vi "Config.View.vi"() -> ()   [LabVIEW 2019]
uses:
  Telas.ctl
  <vilib>/Utility/miscctls.llb/LVPositionTypeDef.ctl
  <vilib>/Utility/miscctls.llb/LVPointTypeDef.ctl
  TelaConfig/Configuracao.Variaveis.vi
panel:
  in  "NovaSenhaOk":bool
  out "SemSenha":bool
  out "SenhaCadastrada":i32[](array[numeric])
  out "ProximaTela":T1
  in  "Tab":enum32{"Page 1", "Page 2"}(tab)
  in  "Salvar":bool
  in  "TabTela":enum32{"Senha", "Campos1", "Campos2"}(tab)
  in  "NextSenha":bool
  out "AlertaSenha":string
  in  "Senha":string caption="SENHA"
  out "TexSegundo":string
  in  "ProximaTela":bool
  in  "AddParametro":bool caption="Adicionar:"
  in  "ListParamentos":string[][](table)
  in  "MeCompleta":bool caption="Memória completa:"
  in  "PosiçaoMemoria":dbl caption="Posiçao na memória:"
  out "TexBit":string
  in  "TamanhoMemoria":enum16{"1 bit", "8 bit", "16 bit"}(ring) caption="Tamanho:"
  in  "TipoMemoria":enum16{"Int", "Boleano"}(ring) caption="Tipo:"
  in  "Memoria":string caption="Memória:"
  in  "AceleracaoMaxima":dbl caption="Tempo mím aceleração:"
  in  "ModeloInversor":string caption="Modelo:"
  out "TexInversor":string
  in  "Parametros":T2(ring) caption="Parâmetros:"
  out "TexMotor":string
  in  "RotacaoMaxMotor":dbl caption="Rotação máxima:"
  in  "PotenciaMotor":dbl caption="Potência:"
  in  "ModeloMotor":string caption="Modelo:"
  in  "NovaSenha":string caption="Nova senha:"
  in  "SelecaoMudaSenha":bool
  out "TexSenha":string
  in  "TaxaComunicSerial":u32 caption="Taxa de comunicação serial:"
  in  "PortaCom":refnum<visa-resource-name> caption="Porta COM:"
  in  "VoltarTela":bool
  out "TexComunic":string
  in  "Paridade":enum16{"Nenhuma", "Ímpar", "Par"}(ring) caption="Paridade:"
  in  "EnderecoSerial":u8 caption="Endereço serial:"
  in  "MudarSenha":bool caption="Mudar:"
  in  "SenhaAntiga":string caption="Senha antiga:"
  out "StatusMudaSenha":string
  in  "Voltar":bool
  out "InfoConfig":string
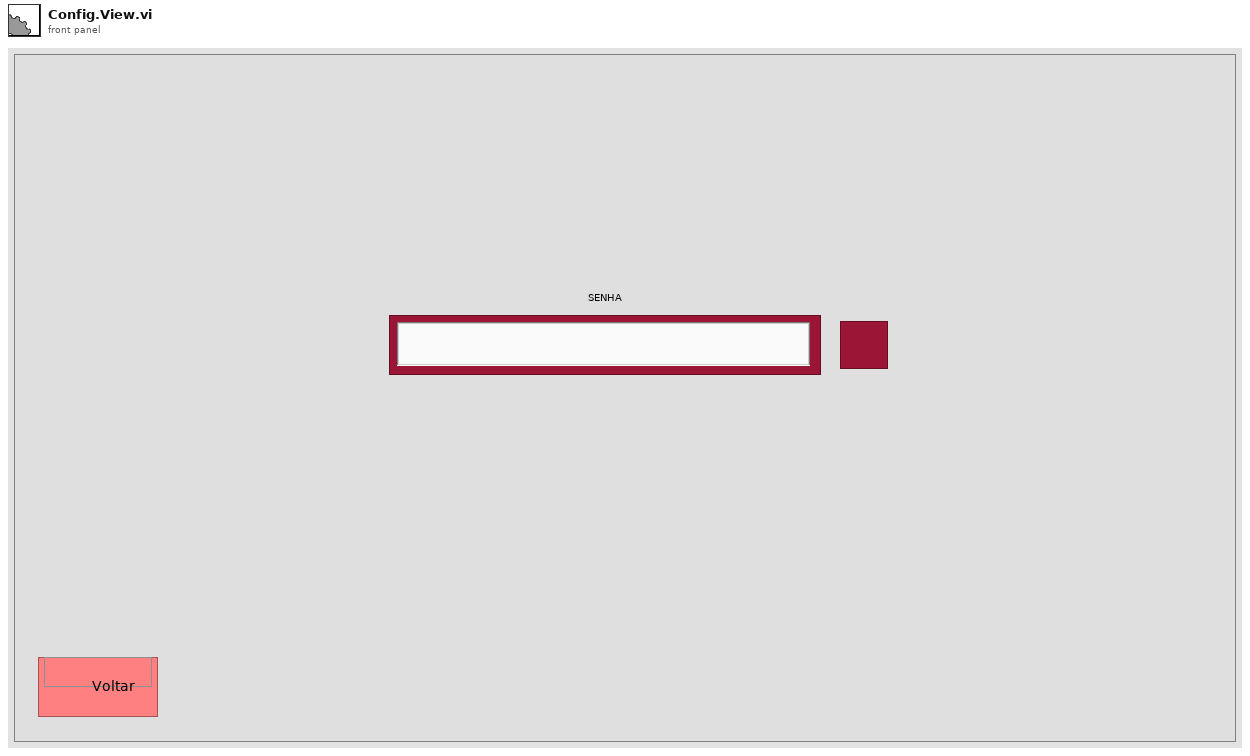
[diagram p1: front panel]
types:
  T1 = typedef "Telas.ctl" = enum16{"Selecao", "Config", "Medicao", "ParametrosTeste"}
  T2 = enum16{"None", "Em Alarme (Leitura)", "Status habilita geral (Leitura)", "Sentido de giro (Leitura)", "Status Remoto (Leitura)", "Em Falha (Leitura)", "Velocidade atual (Leitura)", "Gira/Para (Escrita)", "Habilitar (Escrita)", "Sentido de giro (Escrita) ", "Modo remoto (Escrita)", "Reset falhas (Escrita)", "Referência de velocidade (Escrita)"}
  T3 = typedef "LVPositionTypeDef.ctl" = cluster{"Left":i32, "Top":i32}
  T4 = typedef "LVPointTypeDef.ctl" = cluster{"Horizontal":i16, "Vertical":i16}
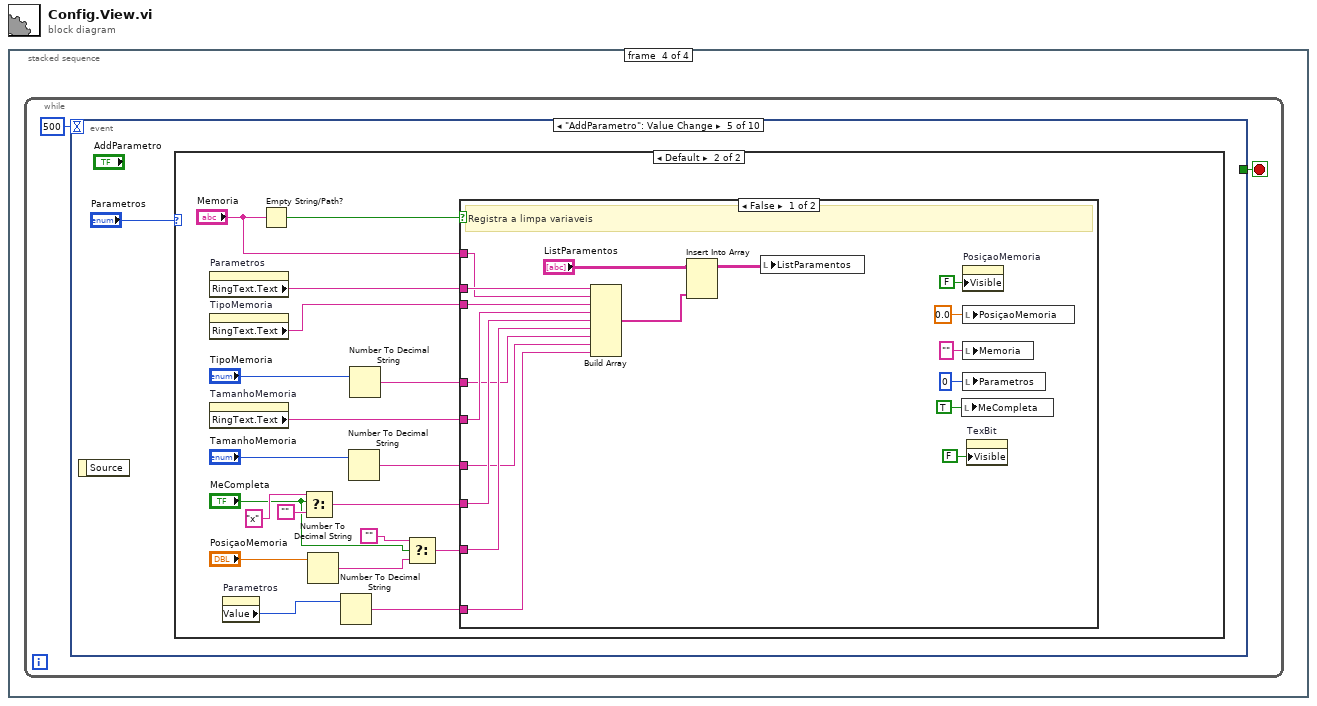
[diagram p0: block diagram]
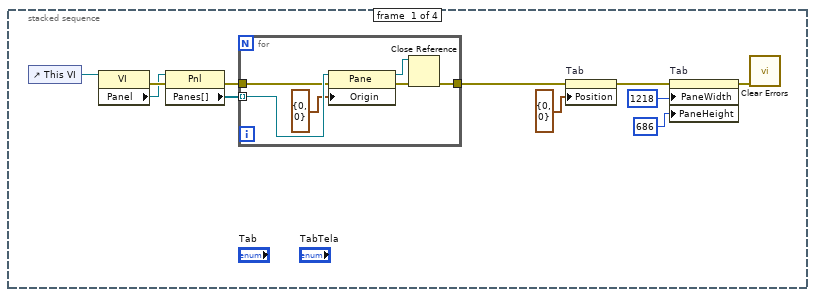
[diagram p2: hidden frame]
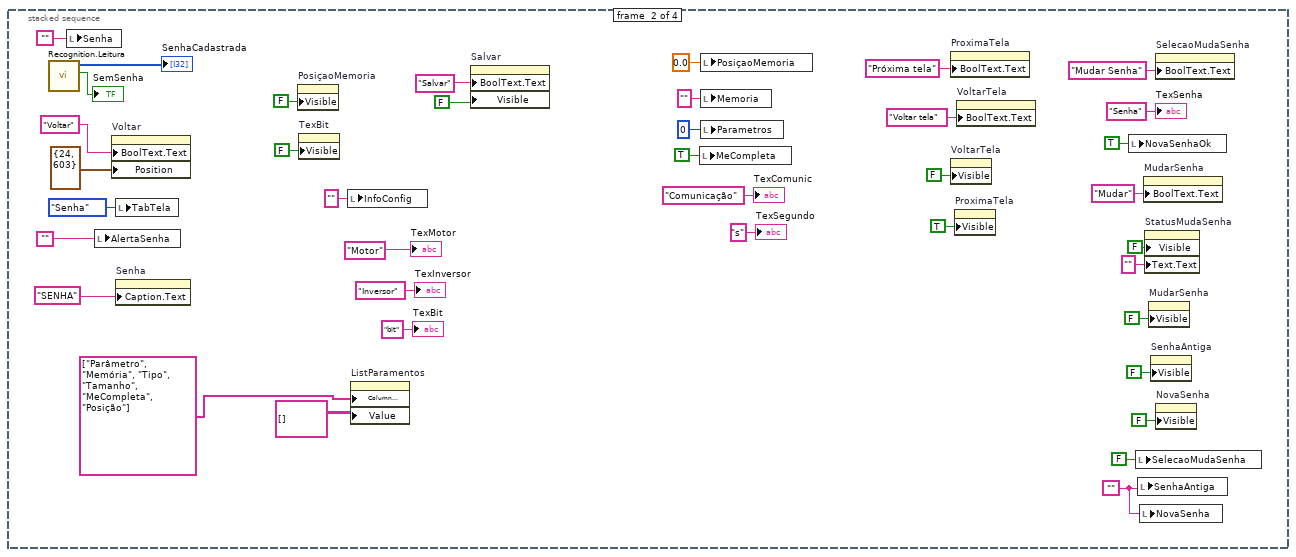
[diagram p3: hidden frame]
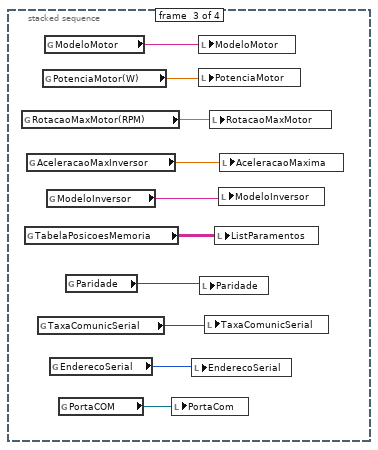
[diagram p4: hidden frame]
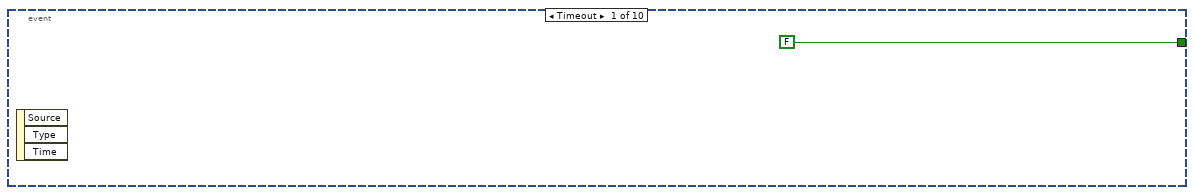
[diagram p5: hidden frame]
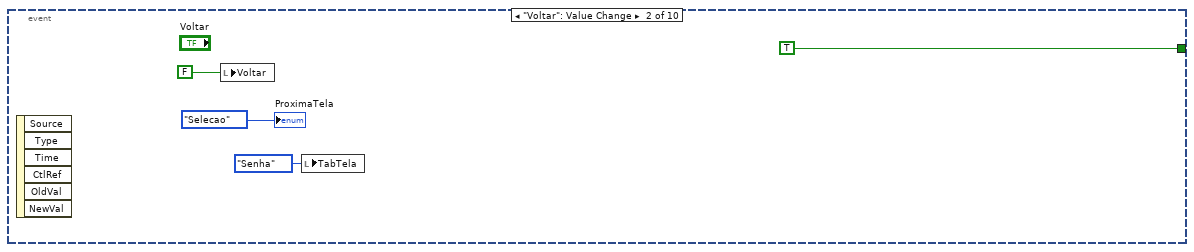
[diagram p6: hidden frame]
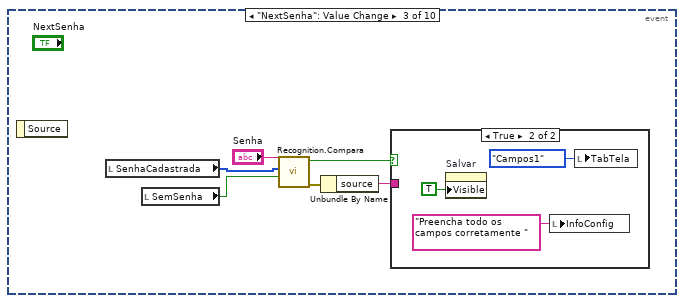
[diagram p7: hidden frame]
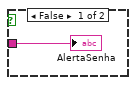
[diagram p8: hidden frame]
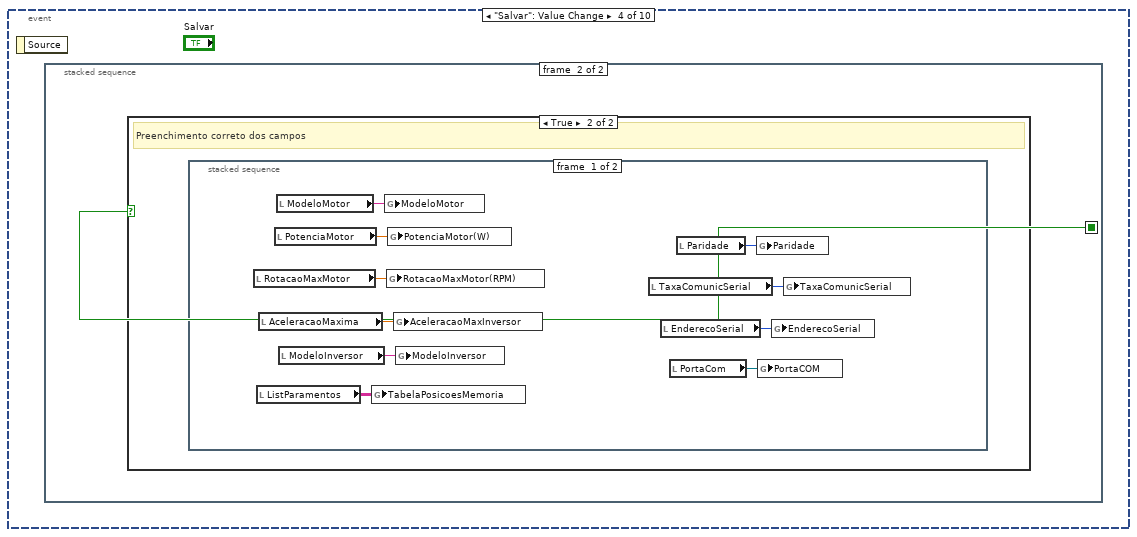
[diagram p9: hidden frame]
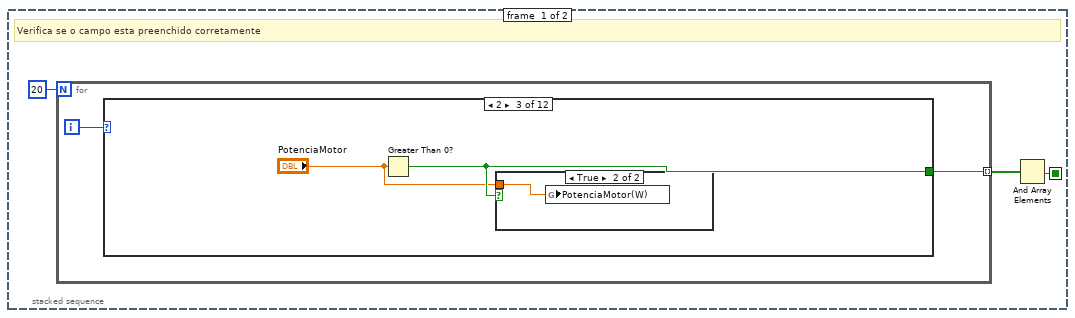
[diagram p10: hidden frame]
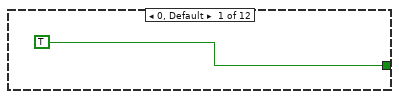
[diagram p11: hidden frame]
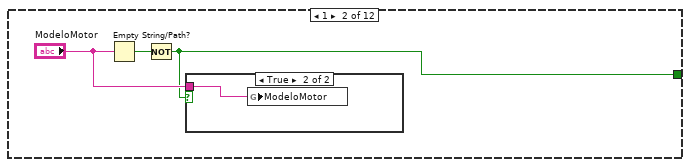
[diagram p12: hidden frame]
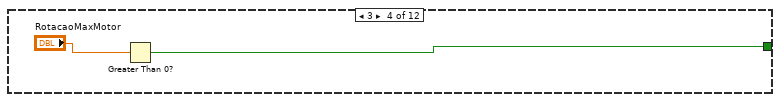
[diagram p15: hidden frame]
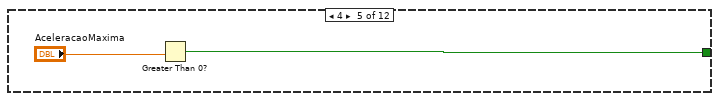
[diagram p16: hidden frame]
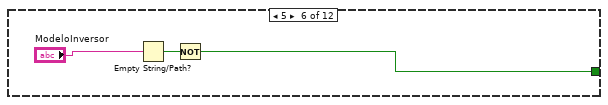
[diagram p17: hidden frame]
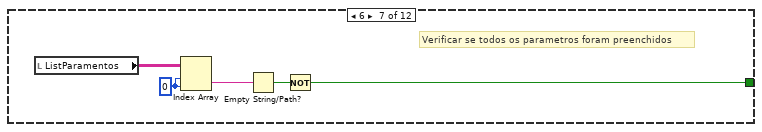
[diagram p18: hidden frame]
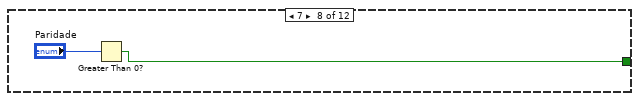
[diagram p19: hidden frame]
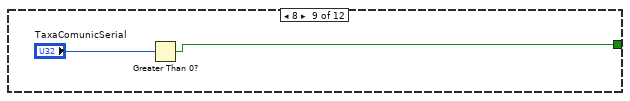
[diagram p20: hidden frame]
diagram:
  n1 = stacked-sequence {
    frame #0 {
      n2 = control-ref of="This VI"() -> (w8:refnum<vi>)
      n3 = property class="VI"(reference=w8) -> (error out=w11:errorcluster, "Panel"=w10:refnum<vi>)  [unwired: 1 in, 1 out]
      n4 = property class="Pnl"(reference=w10, error in=w11) -> (error out=w7:errorcluster, "Panes[]"=w9:refnum<vi>[])  [unwired: 1 out]
      n5 = for {
        tunnel: w9 -> [w17] mode=indexing
        tunnel: w7 -> [w13]
        tunnel: [w12] -> w6
        n6 = property class="Pane"(reference=w17, error in=w13, "Origin"=T4 {"Horizontal"=0, "Vertical"=0}) -> (reference out=w14:refnum<vi>, error out=w15:errorcluster)
        n7 = Close Reference(reference=w14, error in (no error)=w15) -> (error out=w12:errorcluster)
      }
      n8 = property on="Tab" class="TabCtl (strict)"(error in=w6, "Position"=T3 {"Left"=0, "Top"=0}) -> (error out=w5:errorcluster)  [unwired: 1 in, 1 out]
      n9 = property on="Tab" class="TabCtl (strict)"(error in=w5, "PaneWidth"=u32 1218 ("Tab Control Pane Dimension:Width"), "PaneHeight"=u32 686 ("Tab Control Pane Dimension:Height")) -> (error out=w4:errorcluster)  [unwired: 1 in, 1 out]
      n10 = call <vilib>:"Clear Errors.vi"("error in (no error)"=w4) -> ()  [unwired: 5 in, 2 out]
    }
    frame #1 {
      w19 = ""
      n11 = call "Recognition.Leitura.vi"() -> ("SemSenha"=→"SemSenha":bool, "Senha"=→"SenhaCadastrada":i32[])  [unwired: 9 in, 1 out]
      n12 = local write "Senha"("") -> ()
      n13 = local write "AlertaSenha"("") -> ()
      n14 = property on="Voltar" class="Bool (strict)"("BoolText.Text"="Voltar" ("Boolean Text.Text"), "Position"=T3 {"Left"=24, "Top"=603}) -> ()  [unwired: 2 in, 2 out]
      n15 = local write "TabTela"(enum32{"Senha", "Campos1", "Campos2"}."Senha" ("TabTela")) -> ()
      n16 = property on="Senha" class="Str"("Caption.Text"="SENHA") -> ()  [unwired: 2 in, 2 out]
      n17 = property on="PosiçaoMemoria" class="DigNum (strict)"("Visible"=FALSE) -> ()  [unwired: 2 in, 2 out]
      n18 = property on="TexBit" class="Str"("Visible"=FALSE) -> ()  [unwired: 2 in, 2 out]
      n19 = local write "InfoConfig"("" ("InfoConfig")) -> ()
      n20 = property on="ListParamentos" class="Tbl (strict)"("Column Headers[]"=string[] ["Parâmetro", "Memória", "Tipo", "Tamanho", "MeCompleta", "Posição"] ("Column Header Strings[]"), "Value"=string[][] [] ("Item Names")) -> ()  [unwired: 2 in, 2 out]
      n21 = property on="Salvar" class="Bool"("BoolText.Text"="Salvar" ("Boolean Text.Text"), "Visible"=FALSE) -> ()  [unwired: 2 in, 2 out]
      n22 = local write "MeCompleta"(TRUE ("MempriaCompleta")) -> ()
      n23 = local write "PosiçaoMemoria"(0.0 ("PosiçaoMemoria")) -> ()
      n24 = local write "Memoria"("" ("Memoria")) -> ()
      n25 = local write "Parametros"(0) -> ()
      n26 = property on="ProximaTela" class="Bool"("BoolText.Text"="Próxima tela" ("Boolean Text.Text")) -> ()  [unwired: 2 in, 2 out]
      n27 = property on="VoltarTela" class="Bool"("Visible"=FALSE) -> ()  [unwired: 2 in, 2 out]
      n28 = property on="ProximaTela" class="Bool"("Visible"=TRUE) -> ()  [unwired: 2 in, 2 out]
      n29 = property on="VoltarTela" class="Bool"("BoolText.Text"="Voltar tela" ("Boolean Text.Text")) -> ()  [unwired: 2 in, 2 out]
      n30 = local write "NovaSenhaOk"(TRUE ("NovaSenhaOk")) -> ()
      n31 = local write "SelecaoMudaSenha"(FALSE ("SelecaoMudaSenha")) -> ()
      n32 = local write "SenhaAntiga"(w19) -> ()
      n33 = local write "NovaSenha"(w19) -> ()
      n34 = property on="MudarSenha" class="Bool"("BoolText.Text"="Mudar" ("Boolean Text.Text")) -> ()  [unwired: 2 in, 2 out]
      n35 = property on="StatusMudaSenha" class="Str"("Visible"=FALSE, "Text.Text"="") -> ()  [unwired: 2 in, 2 out]
      n36 = property on="MudarSenha" class="Bool"("Visible"=FALSE) -> ()  [unwired: 2 in, 2 out]
      n37 = property on="SenhaAntiga" class="Str"("Visible"=FALSE) -> ()  [unwired: 2 in, 2 out]
      n38 = property on="SelecaoMudaSenha" class="Bool (strict)"("BoolText.Text"="Mudar Senha" ("Boolean Text.Text")) -> ()  [unwired: 2 in, 2 out]
      n39 = property on="NovaSenha" class="Str"("Visible"=FALSE) -> ()  [unwired: 2 in, 2 out]
      "TexMotor" <- "Motor" ("TexMotor")
      "TexInversor" <- "Inversor" ("TexInversor")
      "TexBit" <- "bit" ("TexBit")
      "TexComunic" <- "Comunicação" ("TexConfigComunic")
      "TexSenha" <- "Senha" ("TexSenha")
      "TexSegundo" <- "s" ("TexSegundo")
    }
    frame #2 {
      n40 = global read "Configuracao.Variaveis.vi" "RotacaoMaxMotor(RPM)"() -> (w64:dbl)
      n41 = global read "Configuracao.Variaveis.vi" "TabelaPosicoesMemoria"() -> (w61:string[][])
      n42 = global read "Configuracao.Variaveis.vi" "AceleracaoMaxInversor"() -> (w63:dbl)
      n43 = global read "Configuracao.Variaveis.vi" "TaxaComunicSerial"() -> (w58:u32)
      n44 = global read "Configuracao.Variaveis.vi" "PotenciaMotor(W)"() -> (w65:dbl)
      n45 = global read "Configuracao.Variaveis.vi" "ModeloMotor"() -> (w66:string)
      n46 = global read "Configuracao.Variaveis.vi" "ModeloInversor"() -> (w62:string)
      n47 = global read "Configuracao.Variaveis.vi" "EnderecoSerial"() -> (w59:u8)
      n48 = global read "Configuracao.Variaveis.vi" "PortaCOM"() -> (w60:refnum<visa-resource-name>)
      n49 = global read "Configuracao.Variaveis.vi" "Paridade"() -> (w57:u16)
      n50 = local write "PortaCom"(w60) -> ()
      n51 = local write "EnderecoSerial"(w59) -> ()
      n52 = local write "ModeloMotor"(w66) -> ()
      n53 = local write "PotenciaMotor"(w65) -> ()
      n54 = local write "Paridade"(w57) -> ()
      n55 = local write "TaxaComunicSerial"(w58) -> ()
      n56 = local write "RotacaoMaxMotor"(w64) -> ()
      n57 = local write "ListParamentos"(w61) -> ()
      n58 = local write "ModeloInversor"(w62) -> ()
      n59 = local write "AceleracaoMaxima"(w63) -> ()
    }
    frame #3 {
      n60 = while {
        stop <- w67 stop-if-true
        n61 = event shown="[4] \"AddParametro\": Value Change" {
          selector: _ -> [_ _ _ _ _ _ _ _ _ _]
          dyn-events: _ -> [_ _ _ _ _ _ _ _ _ _]
          timeout: 500 -> [_ _ _ _ _ _ _ _ _ _]
          tunnel: [FALSE TRUE _ _ _ _ _ _ _ _] -> w67
          event Timeout {
            n62 = event-data() -> ()  [unwired: 1 in, 3 out]
          }
          event "Voltar": Value Change {
            n63 = event-data() -> ()  [unwired: 1 in, 6 out]
            n64 = local write "Voltar"(FALSE ("VoltarButton")) -> ()
            n65 = local write "TabTela"(enum32{"Senha", "Campos1", "Campos2"}."Senha" ("TabTela")) -> ()
            "ProximaTela" <- Telas."Selecao" ("NextScreen")
          }
          event "NextSenha": Value Change {
            n66 = event-data() -> ()  [unwired: 1 in, 1 out]
            n67 = local read "SenhaCadastrada"() -> (w78:i32[])
            n68 = local read "SemSenha"() -> (w77:bool)
            n69 = call "Recognition.Compara.vi"("SemSenha"=w77, "SenhaCadastrada"=w78, "Senha"="Senha") -> ("error out"=w76:errorcluster, "SenhaOk"=w74:bool)  [unwired: 7 in]
            n70 = Unbundle By Name(w76) -> ("source"=w75:string)
            n71 = case shown="True" w74 {
              tunnel: w75 -> [w80 _]
              frame False {
                "AlertaSenha" <- w80
              }
              frame True {
                n72 = property on="Salvar" class="Bool"("Visible"=TRUE) -> ()  [unwired: 2 in, 2 out]
                n73 = local write "InfoConfig"("Preencha todo os campos corretamente " ("InfoConfig")) -> ()
                n74 = local write "TabTela"(enum32{"Senha", "Campos1", "Campos2"}."Campos1" ("TabTela")) -> ()
              }
            }
          }
          event "Salvar": Value Change {
            n75 = event-data() -> ()  [unwired: 1 in, 1 out]
            n76 = stacked-sequence {
              seq-local: [w84 _] -> [_ w119]
              frame #0 {
                # "Verifica se o campo esta preenchido corretamente"
                n77 = for {
                  N: 20 -> [_]
                  tunnel: [w87] -> w85 mode=indexing
                  i -> [w88]
                  n78 = case shown="2" w88 {
                    tunnel: [TRUE w90 w95 w97 w99 w102 w104 w109 w111 w113 w115 "NovaSenhaOk"] -> w87
                    frame 0, Default {
                    }
                    frame 1 {
                      n79 = Empty String/Path?(string/path="ModeloMotor") -> (empty?=w92:bool)
                      n80 = Not(x=w92) -> (.not. x?=w90:bool)
                      n81 = case shown="True" w90 {
                        tunnel: "ModeloMotor" -> [_ w93]
                        frame False {
                        }
                        frame True {
                          n82 = global write "Configuracao.Variaveis.vi" "ModeloMotor"(w93) -> ()
                        }
                      }
                    }
                    frame 2 {
                      n83 = Greater Than 0?(x="PotenciaMotor") -> (x > 0?=w95:bool)
                      n84 = case shown="True" w95 {
                        tunnel: "PotenciaMotor" -> [_ w96]
                        frame False {
                        }
                        frame True {
                          n85 = global write "Configuracao.Variaveis.vi" "PotenciaMotor(W)"(w96) -> ()
                        }
                      }
                    }
                    frame 3 {
                      n86 = Greater Than 0?(x="RotacaoMaxMotor") -> (x > 0?=w97:bool)
                    }
                    frame 4 {
                      n87 = Greater Than 0?(x="AceleracaoMaxima") -> (x > 0?=w99:bool)
                    }
                    frame 5 {
                      n88 = Empty String/Path?(string/path="ModeloInversor") -> (empty?=w103:bool)
                      n89 = Not(x=w103) -> (.not. x?=w102:bool)
                    }
                    frame 6 {
                      w107 = 0 ("disabled index (col)")
                      # "Verificar se todos os parametros foram preenchidos"
                      n90 = local read "ListParamentos"() -> (w108:string[][])
                      n91 = Index Array(array=w108, index (row)=w107, index (col)=w107) -> (element=w105:string)
                      n92 = Empty String/Path?(string/path=w105) -> (empty?=w106:bool)
                      n93 = Not(x=w106) -> (.not. x?=w104:bool)
                    }
                    frame 7 {
                      n94 = Greater Than 0?(x="Paridade") -> (x > 0?=w109:bool)
                    }
                    frame 8 {
                      n95 = Greater Than 0?(x="TaxaComunicSerial") -> (x > 0?=w111:bool)
                    }
                    frame 9 {
                      n96 = Greater Than 0?(x="EnderecoSerial") -> (x > 0?=w113:bool)
                    }
                    frame 10 {
                      n97 = Empty String/Path?(string/path="PortaCom") -> (empty?=w117:bool)
                      n98 = Not(x=w117) -> (.not. x?=w115:bool)
                    }
                    frame 11 {
                    }
                  }
                }
                n99 = And Array Elements(Boolean array=w85) -> (logical AND=w84:bool)
              }
              frame #1 {
                n100 = case shown="True" w119 {
                  frame False {
                    # "Algo não esta preenchido corretamente"
                    "InfoConfig" <- "Erro: Falta preencher algum campo corretamente" ("InfoConfig")
                  }
                  frame True {
                    # "Preenchimento correto dos campos"
                    n101 = stacked-sequence {
                      frame #0 {
                        n102 = local read "RotacaoMaxMotor"() -> (w126:dbl)
                        n103 = local read "ListParamentos"() -> (w129:string[][])
                        n104 = local read "AceleracaoMaxima"() -> (w127:dbl)
                        n105 = local read "PotenciaMotor"() -> (w125:dbl)
                        n106 = local read "ModeloMotor"() -> (w130:string)
                        n107 = local read "ModeloInversor"() -> (w128:string)
                        n108 = global write "Configuracao.Variaveis.vi" "TabelaPosicoesMemoria"(w129) -> ()
                        n109 = global write "Configuracao.Variaveis.vi" "ModeloMotor"(w130) -> ()
                        n110 = global write "Configuracao.Variaveis.vi" "RotacaoMaxMotor(RPM)"(w126) -> ()
                        n111 = global write "Configuracao.Variaveis.vi" "PotenciaMotor(W)"(w125) -> ()
                        n112 = global write "Configuracao.Variaveis.vi" "AceleracaoMaxInversor"(w127) -> ()
                        n113 = global write "Configuracao.Variaveis.vi" "ModeloInversor"(w128) -> ()
                        n114 = local read "TaxaComunicSerial"() -> (w123:u32)
                        n115 = local read "EnderecoSerial"() -> (w122:u8)
                        n116 = local read "PortaCom"() -> (w121:refnum<visa-resource-name>)
                        n117 = local read "Paridade"() -> (w124:enum16{"Nenhuma", "Ímpar", "Par"})
                        n118 = global write "Configuracao.Variaveis.vi" "Paridade"(w124) -> ()
                        n119 = global write "Configuracao.Variaveis.vi" "PortaCOM"(w121) -> ()
                        n120 = global write "Configuracao.Variaveis.vi" "EnderecoSerial"(w122) -> ()
                        n121 = global write "Configuracao.Variaveis.vi" "TaxaComunicSerial"(w123) -> ()
                      }
                      frame #1 {
                        n122 = call "Configuracao.Escrita.vi"() -> ("error out"=w131:errorcluster)  [unwired: 11 in]
                        n123 = case shown="No Error" w131 {
                          tunnel: ["Informações salvas" ("InfoConfig") "Erro ao salvar as variavies" ("InfoConfig")] -> w132
                          frame No Error {
                          }
                          frame Error {
                          }
                        }
                        n124 = local write "InfoConfig"(w132) -> ()
                      }
                    }
                  }
                }
              }
            }
          }
          event "AddParametro": Value Change {
            n125 = event-data() -> ()  [unwired: 1 in, 1 out]
            n126 = case shown="Default" "Parametros" {
              frame "None" {
                # "Sem seleção de parametro. Erro"
              }
              frame Default {
                n127 = property on="Parametros" class="Enum (strict)"() -> ("RingText.Text"=w149:string)  [unwired: 2 in, 2 out]
                n128 = property on="TipoMemoria" class="Enum (strict)"() -> ("RingText.Text"=w148:string)  [unwired: 2 in, 2 out]
                n129 = property on="TamanhoMemoria" class="Enum (strict)"() -> ("RingText.Text"=w147:string)  [unwired: 2 in, 2 out]
                n130 = property on="Parametros" class="Enum (strict)"() -> ("Value"=w137:T2)  [unwired: 2 in, 2 out]
                n131 = Empty String/Path?(string/path="Memoria") -> (empty?=w154:bool)
                n132 = Select(t="x", s="MeCompleta", f="") -> (s? t:f=w146:string)
                n133 = Number To Decimal String(number="PosiçaoMemoria") -> (decimal integer string=w143:string)  [unwired: 1 in]
                n134 = Number To Decimal String(number=w137) -> (decimal integer string=w136:string)  [unwired: 1 in]
                n135 = Number To Decimal String(number="TamanhoMemoria") -> (decimal integer string=w138:string)  [unwired: 1 in]
                n136 = Number To Decimal String(number="TipoMemoria") -> (decimal integer string=w140:string)  [unwired: 1 in]
                n137 = Select(t="", s="MeCompleta", f=w143) -> (s? t:f=w142:string)
                n138 = case shown="False" w154 {
                  tunnel: "Memoria" -> [w171 _]
                  tunnel: w149 -> [w172 _]
                  tunnel: w148 -> [w170 _]
                  tunnel: w147 -> [w169 _]
                  tunnel: w146 -> [w168 _]
                  tunnel: w142 -> [w167 _]
                  tunnel: w140 -> [w166 _]
                  tunnel: w138 -> [w165 _]
                  tunnel: w136 -> [w155 _]
                  frame False {
                    # "Registra a limpa variaveis"
                    n139 = Build Array(w172, w171, w170, w169, w168, w167, w166, w165, w155) -> (w163:string[])
                    n140 = Insert Into Array(array="ListParamentos", new element=w163) -> (w162:string[][])  [unwired: 2 in]
                    n141 = local write "ListParamentos"(w162) -> ()
                    n142 = local write "MeCompleta"(TRUE ("MempriaCompleta")) -> ()
                    n143 = property on="PosiçaoMemoria" class="DigNum (strict)"("Visible"=FALSE) -> ()  [unwired: 2 in, 2 out]
                    n144 = local write "PosiçaoMemoria"(0.0 ("PosiçaoMemoria")) -> ()
                    n145 = local write "Memoria"("" ("Memoria")) -> ()
                    n146 = local write "Parametros"(0) -> ()
                    n147 = property on="TexBit" class="Str"("Visible"=FALSE) -> ()  [unwired: 2 in, 2 out]
                  }
                  frame True {
                    # "Memoria vazia. Erro"
                  }
                }
              }
            }
          }
          event "MeCompleta": Value Change {
            n148 = event-data() -> ()  [unwired: 1 in, 1 out]
            n149 = local read "MeCompleta"() -> (w174:bool)
            n150 = Not(x=w174) -> (.not. x?=w173:bool)
            n151 = property on="PosiçaoMemoria" class="DigNum (strict)"("Visible"=w173) -> ()  [unwired: 2 in, 2 out]
            n152 = property on="TexBit" class="Str"("Visible"=w173) -> ()  [unwired: 2 in, 2 out]
          }
          event "ProximaTela": Value Change {
            n153 = event-data() -> ()  [unwired: 1 in, 1 out]
            n154 = local write "TabTela"(enum32{"Senha", "Campos1", "Campos2"}."Campos2" ("TabTela")) -> ()
            n155 = property on="VoltarTela" class="Bool"("Visible"=TRUE) -> ()  [unwired: 2 in, 2 out]
            n156 = property on="ProximaTela" class="Bool"("Visible"=FALSE) -> ()  [unwired: 2 in, 2 out]
          }
          event "SelecaoMudaSenha": Value Change {
            n157 = event-data() -> ()  [unwired: 1 in, 6 out]
            n158 = property on="MudarSenha" class="Bool"("Visible"="SelecaoMudaSenha") -> ()  [unwired: 2 in, 2 out]
            n159 = property on="SenhaAntiga" class="Str"("Visible"="SelecaoMudaSenha") -> ()  [unwired: 2 in, 2 out]
            n160 = property on="NovaSenha" class="Str"("Visible"="SelecaoMudaSenha") -> ()  [unwired: 2 in, 2 out]
            n161 = Not(x="SelecaoMudaSenha") -> (.not. x?=w180:bool)
            n162 = property on="StatusMudaSenha" class="Str"("Visible"="SelecaoMudaSenha") -> ()  [unwired: 2 in, 2 out]
            n163 = local write "NovaSenhaOk"(w180) -> ()
            n164 = local write "StatusMudaSenha"("" ("StatusMudaSenha")) -> ()
          }
          event "VoltarTela": Value Change {
            n165 = event-data() -> ()  [unwired: 1 in, 6 out]
            n166 = local write "TabTela"(enum32{"Senha", "Campos1", "Campos2"}."Campos1" ("TabTela")) -> ()
            n167 = property on="VoltarTela" class="Bool"("Visible"=FALSE) -> ()  [unwired: 2 in, 2 out]
            n168 = property on="ProximaTela" class="Bool"("Visible"=TRUE) -> ()  [unwired: 2 in, 2 out]
          }
          event "MudarSenha": Value Change {
            n169 = event-data() -> ()  [unwired: 1 in, 6 out]
            n170 = call "Recognition.Leitura.vi"() -> ("error out"=w184:errorcluster, "SemSenha"=w185:bool, "Senha"=w186:i32[])  [unwired: 9 in]
            n171 = call "Recognition.Compara.vi"("error in"=w184, "SemSenha"=w185, "SenhaCadastrada"=w186, "Senha"="SenhaAntiga") -> ("error out"=w189:errorcluster, "SenhaOk"=w190:bool)  [unwired: 6 in]
            n172 = case shown="True" w190 {
              tunnel: w189 -> [w194 w199]
              tunnel: [w193 w198] -> w188
              tunnel: [FALSE w197] -> w187
              frame False {
                n173 = Unbundle By Name(w194) -> ("source"=w193:string)
              }
              frame True {
                n174 = Empty String/Path?(string/path="NovaSenha") -> (empty?=w195:bool)
                n175 = case shown="True" w195 {
                  tunnel: "NovaSenha" -> [w204 _]
                  tunnel: w199 -> [w203 _]
                  tunnel: [w201 "Adicione uma senha"] -> w198
                  tunnel: [w200 FALSE] -> w197
                  frame False {
                    n176 = call "Recognition.Salva.vi"("error in (no error)"=w203, "Senha"=w204) -> ("error out"=w202:errorcluster)  [unwired: 9 in]
                    n177 = case shown="Error .." w202 {
                      tunnel: ["Senha salva com sucesso" "Erro ao salvar a senha"] -> w201
                      tunnel: [TRUE FALSE] -> w200
                      frame No Error {
                      }
                      frame Error {
                      }
                    }
                  }
                  frame True {
                  }
                }
              }
            }
            "StatusMudaSenha" <- w188
            n178 = local write "NovaSenhaOk"(w187) -> ()
          }
        }
      }
    }
  }
